vi "_skipComments.vi"(8 "error in (no error)":errorcluster, 11 "JSON Parser In":refnum<class "tJSONParser.lvclass">) -> (0 "error out":errorcluster, 3 "JSON Parser Out":refnum<class "tJSONParser.lvclass">)   [LabVIEW 2013, in "JSON.lvlib" / "tJSONParser.lvclass"]
doc: "Consumes all comments. Errors if the comment isn't of the form \"//.*\"."
uses:
  tJSONParser.lvclass
  tJSONParser.lvclass/tJSONParser.ctl
  _error.ctl
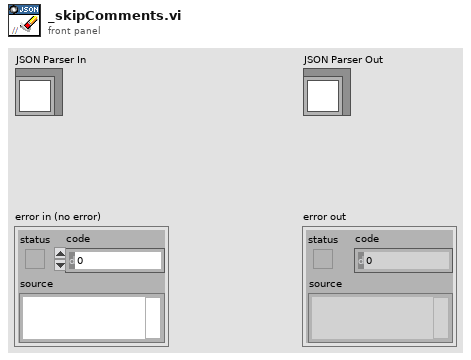
[diagram p1: front panel]
types:
  T1 = typedef "JSON.lvlib/tJSONParser.lvclass/_error.ctl" = enum16{"Missing Object Open", "Missing Pair Separator", "Missing Object End Or Separator", "Missing Pair String", "Unexpected Token", "Missing Array End Or Separator", "Invalid Escape Sequence", "Unexpected End Of File", "Invalid Unicode", "Unexpected End Of Line", "Invalid Numerical Constant"}
  T2 = typedef "JSON.lvlib/tJSONParser.lvclass/_tokenType.ctl" = enum16{"Object Begin", "Object End", "Array Begin", "Array End", "String Delimeter", "Forward Slash", "Number", "Boolean", "Null", "Object Or Array Separator", "Pair Separator", "End Of File", "Asterisk", "Backward Slash", "Other"}
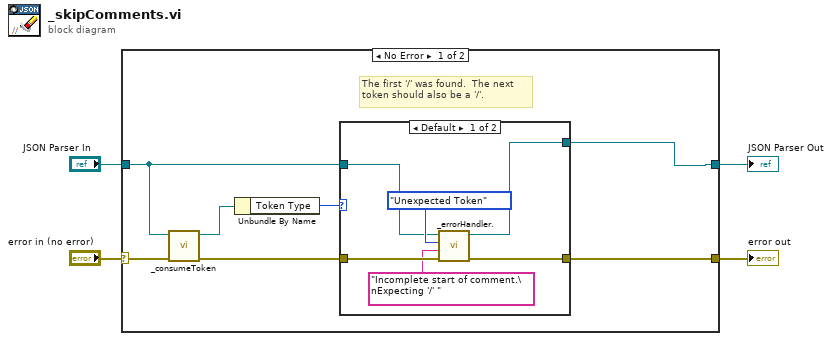
[diagram p0: block diagram]
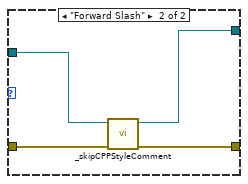
[diagram p2: hidden frame]
diagram:
  n1 = case shown="No Error" "error in (no error)" {
    selector: "error in (no error)" -> [w9 w23]
    tunnel: [w11 w23] -> w3
    tunnel: [w10 w22] -> w2
    tunnel: "JSON Parser In" -> [w7 w22]
    frame No Error {
      # "The first '/' was found.  The next\ntoken should also be a '/'."
      n2 = call "_consumeToken.vi"("error in (no error)"=w9, "JSON Parser In"=w7) -> ("error out"=w8:errorcluster, "JSON Parser Out"=w6:refnum<class "tJSONParser.lvclass">)  [unwired: 8 in]
      n3 = Unbundle By Name(w6) -> ("Token Type"=w5:T2)
      n4 = case shown="Default" w5 {
        tunnel: w8 -> [w17 w21]
        tunnel: [w16 w20] -> w11
        tunnel: w7 -> [w13 w18]
        tunnel: [w12 w19] -> w10
        frame Default {
          n5 = call "_errorHandler..vi"("error in (no error)"=w17, "Additional Text"="Incomplete start of comment.\nExpecting '/' ", "Error Type"=_error."Unexpected Token", "JSON Parser In"=w13) -> ("error out"=w16:errorcluster, "JSON Parser Out"=w12:refnum<class "tJSONParser.lvclass">)  [unwired: 6 in]
        }
        frame "Forward Slash" {
          n6 = call "_skipCPPStyleComment.vi"("error in (no error)"=w21, "JSON Parser In"=w18) -> ("error out"=w20:errorcluster, "JSON Parser Out"=w19:refnum<class "tJSONParser.lvclass">)  [unwired: 8 in]
        }
      }
    }
    frame Error {
    }
  }
  "error out" <- w3
  "JSON Parser Out" <- w2
